vi "catWalkCalibrateServos.vi"() -> ()   [LabVIEW 2012]
panel:
  in  "Servo motor":u16(ring)=1 items=["Gate 0"=0, "Trap"=3, "Sieve"=1, "Ejector"=2]
  in  "stop":bool
  in  "servo custom position":u16(knob)=1000 max=2500 step=10 scale=500.0..2500.0
  in  "gate 0 closed":u16=1390
  in  "fly ejector open":u16=1350
  in  "USB COM port":refnum<visa-resource-name>="COM3"
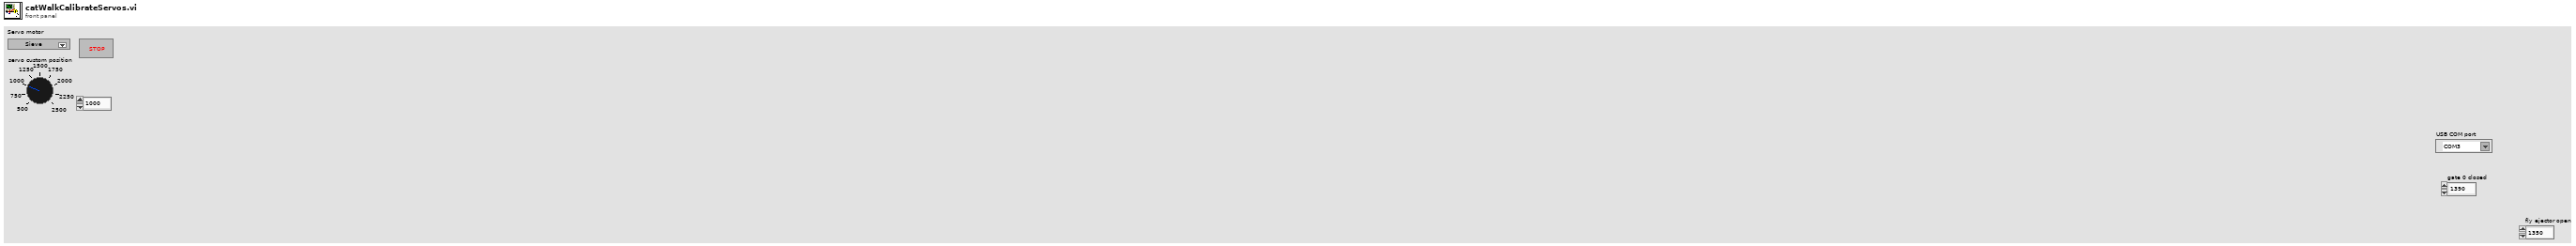
[diagram p1: front panel]
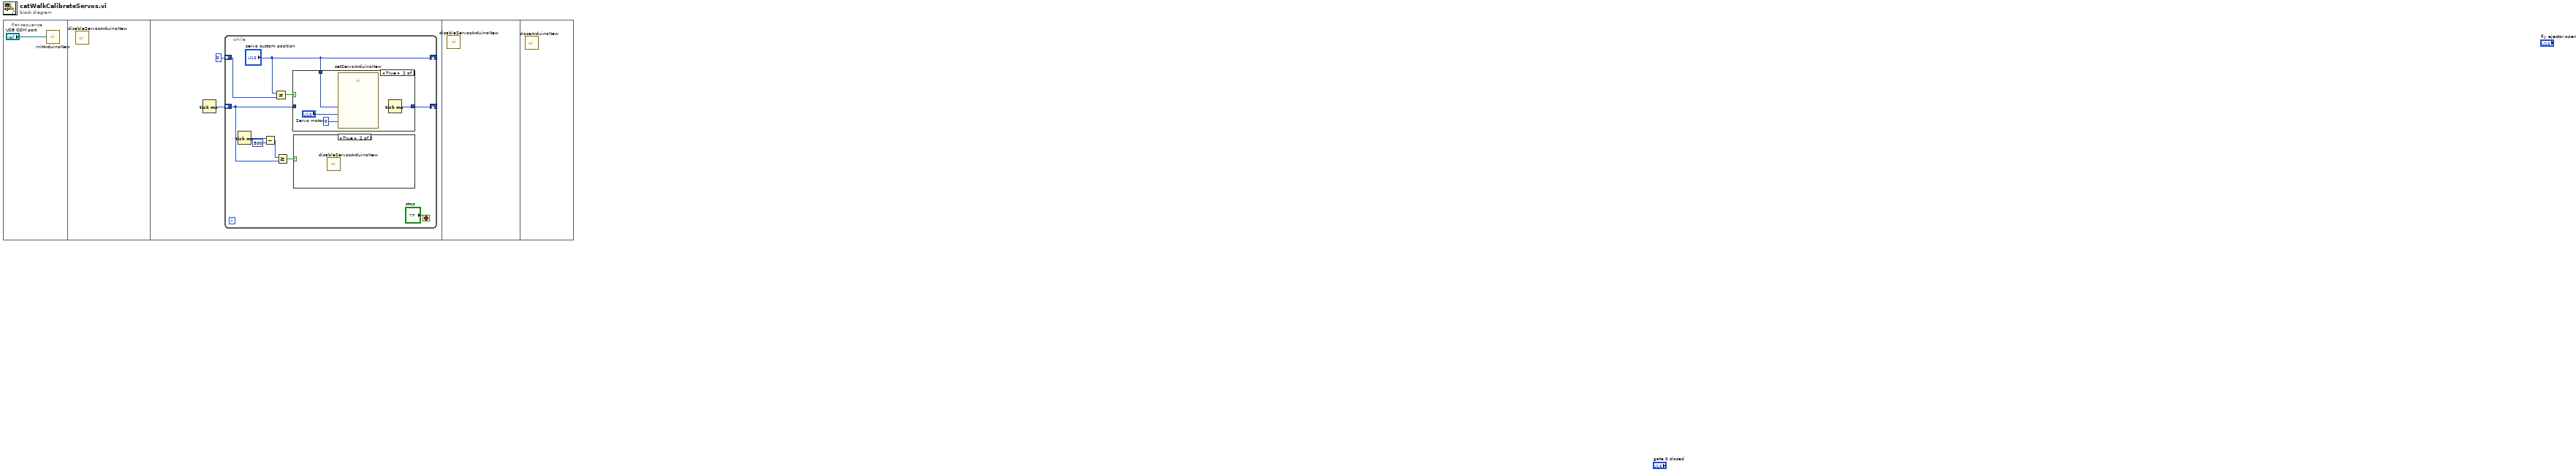
[diagram p0: block diagram]
diagram:
  n1 = flat-sequence {
    frame #0 {
      n2 = call "initArduinoNew.vi"("VISA resource"="USB COM port") -> ()
    }
    frame #1 {
      n3 = call "disableServosArduinoNew.vi"() -> ()  [unwired: 1 in]
    }
    frame #2 {
      n4 = Tick Count (ms)() -> (millisecond timer value=w3:u32)
      n5 = while {
        shift-right: ["servo custom position"] -> _
        shift-left: u16 0 ("servo custom position") -> [w11]
        shift-right: [w10] -> _
        shift-left: w3 -> [w5]
        stop <- "stop" stop-if-true
        n6 = Tick Count (ms)() -> (millisecond timer value=w9:u32)
        n7 = Subtract(x=w9, y=u32 500) -> (x-y=w7:u32)
        n8 = Not Equal?(x="servo custom position", y=w11) -> (x != y?=w12:bool)
        n9 = Greater Or Equal?(x=w7, y=w5) -> (x >= y?=w6:bool)
        n10 = case shown="True" w12 {
          tunnel: "servo custom position" -> [_ w17]
          tunnel: [w14 w16] -> w10
          tunnel: w5 -> [w14 _]
          frame False {
          }
          frame True {
            n11 = call "setServoArduinoNew.vi"("speed"=u8 0, "Pulse Width in uS"=w17, "servo id"="Servo motor") -> ()
            n12 = Tick Count (ms)() -> (millisecond timer value=w16:u32)
          }
        }
        n13 = case shown="True" w6 {
          frame False {
          }
          frame True {
            n14 = call "disableServosArduinoNew.vi"() -> ()  [unwired: 1 in]
          }
        }
      }
    }
    frame #3 {
      n15 = call "disableServosArduinoNew.vi"() -> ()  [unwired: 1 in]
    }
    frame #4 {
      n16 = call "closeArduinoNew.vi"() -> ()  [unwired: 12 in]
    }
  }
